vi "Actor Core.vi"(8 "error in":errorcluster, 11 "My Application":refnum<class "Car Wash Controller.lvclass">) -> (0 "error out":errorcluster, 3 "Actor out":refnum<class "Actor.lvclass">)   [LabVIEW 2012, in "Car Wash Controller.lvlib" / "Car Wash Controller.lvclass"]
doc: "This is Actor Core.vi, the main message handling loop for Actors. An actor usually just sits in this loop and processes messages as they arrive. Any error returned by the message Do.vi call will stop the loop, with error code 43 as the canonical signal to stop with no error sent to caller. Descendants may override that in Handle Error.vi."
uses:
  Car Wash Controller.lvclass
  <vilib>/ActorFramework/Actor/Actor.lvclass
  Simulated Entry Console/Simulated Entry Console/Simulated Entry Console.lvclass
  Simulated Wash Display Console/Simulated Wash Display Console/Simulated Wash Display Console.lvclass
  Vehicle Position Simulation/Vehicle Position Interface Simulation/Vehicle Position Interface Simulation.lvclass
  Simulated Configuration Database/Simulated Configuration Database/Simulated Configuration Database.lvclass
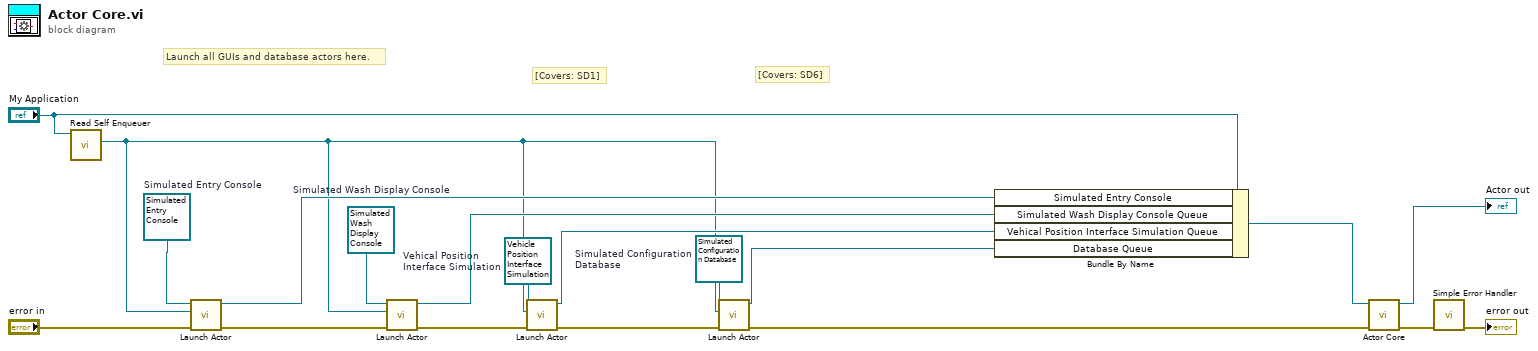
[diagram p0: block diagram]
diagram:
  w4 = refnum<class "Simulated Configuration Database.lvclass"> refnum  # Simulated Configuration Database
  w5 = refnum<class "Vehicle Position Interface Simulation.lvclass"> refnum  # Vehical Position Interface Simulation
  w6 = refnum<class "Simulated Wash Display Console.lvclass"> refnum  # Simulated Wash Display Console
  w7 = refnum<class "Simulated Entry Console.lvclass"> refnum  # Simulated Entry Console
  # "[Covers: SD6]"
  # "[Covers: SD1]"
  # "Launch all GUIs and database actors here."
  n1 = call <vilib>:"Read Self Enqueuer.vi"("Actor"="My Application") -> ("Self Enqueuer"=w1:refnum<class "Message Enqueuer.lvclass">)  [unwired: 10 in]
  n2 = call <vilib>:"Launch Actor.vi"("error in (no error)"="error in", "Actor-to-Caller Enqueuer"=w1, "Actor"=w7) -> ("error out"=w16:errorcluster, "Caller-To-Actor Enqueuer"=w12:refnum<class "Message Enqueuer.lvclass">)  [unwired: 7 in]
  n3 = call <vilib>:"Launch Actor.vi"("error in (no error)"=w16, "Actor-to-Caller Enqueuer"=w1, "Actor"=w6) -> ("error out"=w15:errorcluster, "Caller-To-Actor Enqueuer"=w11:refnum<class "Message Enqueuer.lvclass">)  [unwired: 7 in]
  n4 = call <vilib>:"Launch Actor.vi"("Actor-to-Caller Enqueuer"=w1, "Actor"=w5) -> ("Caller-To-Actor Enqueuer"=w3:refnum<class "Message Enqueuer.lvclass">)  [unwired: 8 in, 1 out]
  n5 = call <vilib>:"Launch Actor.vi"("Actor-to-Caller Enqueuer"=w1, "Actor"=w4) -> ("Caller-To-Actor Enqueuer"=w2:refnum<class "Message Enqueuer.lvclass">)  [unwired: 8 in, 1 out]
  n6 = Bundle By Name(cluster="My Application", "Simulated Entry Console"=w12, "Simulated Wash Display Console Queue"=w11, "Vehical Position Interface Simulation Queue"=w3, "Database Queue"=w2) -> (w13:refnum<class "Car Wash Controller.lvclass">)
  n7 = call-parent "Actor Core.vi"("error in"=w15, "Actor in"=w13) -> ("error out"=w10:errorcluster, "Actor out"=→"Actor out":refnum<class "Actor.lvclass">)  [unwired: 8 in]
  n8 = call <vilib>:"Simple Error Handler.vi"("error in (no error)"=w10) -> ("error out"=→"error out":errorcluster)  [unwired: 4 in, 4 out]
